vi "Ej5b.vi"() -> ()   [LabVIEW 2023]
panel:
  out "Waveform Chart":cluster{"Thermometer":dbl, dbl}(graph)
  in  "stop":bool
  in  "miliseconds delay":dbl(slide) scale=0.0..2000.0
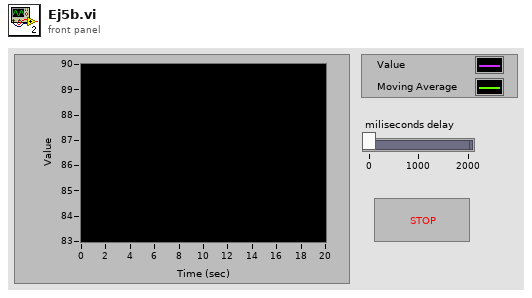
[diagram p1: front panel]
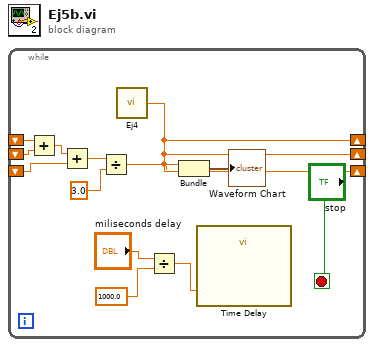
[diagram p0: block diagram]
diagram:
  n1 = while {
    shift-right: [w8] -> _
    shift-left: _ -> [w7]
    shift-right: [w8] -> _
    shift-left: _ -> [w4]
    shift-right: [w8] -> _
    shift-left: _ -> [w6]
    stop <- "stop" stop-if-true
    n2 = Add(x=w7, y=w6) -> (x+y=w5:dbl)
    n3 = Add(x=w5, y=w4) -> (x+y=w3:dbl)
    n4 = Divide(x=w3, y=3.0) -> (x/y=w2:dbl)
    n5 = call "Ej4.vi"() -> ("Thermometer"=w8:dbl)  [unwired: 1 in]
    n6 = Divide(x="miliseconds delay", y=1000.0) -> (x/y=w10:dbl)
    n7 = Bundle("Thermometer"=w8, w2) -> (→"Waveform Chart":cluster{"Thermometer":dbl, dbl})  [unwired: 1 in]
    n8 = call "Time Delay"("Delay Time (s)"=w10) -> ()  [unwired: 10 in, 1 out]
  }
